vi "Write Test Executive Ref.vi"(10 "Test Executive Ref":refnum<data-value>, 11 "Test Executive in":refnum<class "Test Executive.lvclass">) -> (3 "Test Executive out":refnum<class "Test Executive.lvclass">)   [LabVIEW 2017, in "Test Executive.lvlib" / "Test Executive.lvclass"]
uses:
  <vilib>/gpm_packages/@cs/test-executive/Source/Test Executive/TestExecutive/Test Executive.lvclass
  <vilib>/gpm_packages/@cs/linked-list/Source/Linked List/ILinkedList/ILinked List.lvclass
  <vilib>/gpm_packages/@cs/test-executive/Source/Test Executive/TestExecutive/Test Executive.lvclass/Test Executive.ctl
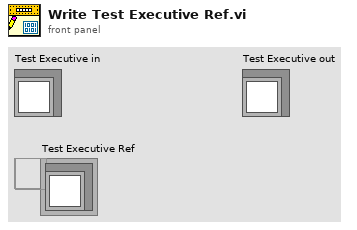
[diagram p1: front panel]
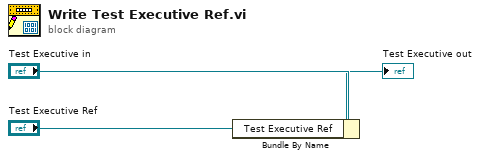
[diagram p0: block diagram]
diagram:
  n1 = Bundle By Name(cluster="Test Executive in", "Test Executive Ref"="Test Executive Ref") -> (→"Test Executive out":refnum<class "Test Executive.lvclass">)
